vi "Interne Werte.vi"(0 "Regler Interne Werte":T2, 1 "Index":i32, 11 "error in (no error)":errorcluster caption="Fehler (Eingang, kein Fehler)", 12 "Aktionen Interne Werte":T1) -> (3 "Änderung?":bool, 4 "FT-IR":sgl[](array[numeric]), 6 "Ausgang":sgl[](array[numeric]), 8 "Dichtheitstest":sgl[](array[numeric]), 10 "Pumpe":sgl[](array[numeric]), 14 "error out":errorcluster caption="Fehler (Ausgang)", 15 "Druck Kalter Block":sgl[](array[numeric]))   [LabVIEW 2020, in "Regler.lvlib" / "Druckregler.lvlib"]
uses:
  Druckregler.lvlib
  Regler Interne Werte.ctl
  Aktionen Interne Werte.ctl
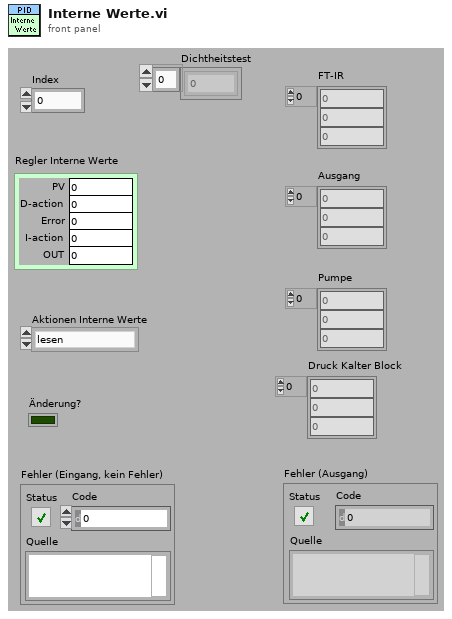
[diagram p1: front panel]
types:
  T1 = typedef "Regler.lvlib/Druckregler.lvlib/Aktionen Interne Werte.ctl" = enum16{"lesen", "FT-IR", "Ausgang", "Pumpe", "laden", "speichern", "Änderung?", "Druck Kalter Block", "Dichtheitstest"}
  T2 = typedef "Regler.lvlib/Druckregler.lvlib/Regler Interne Werte.ctl" = cluster{"PV":sgl, "D-action":sgl, "Error":sgl, "I-action":sgl, "OUT":sgl}
  T3 = cluster{sgl[][], sgl[][], sgl[][], sgl[][], sgl[][]}
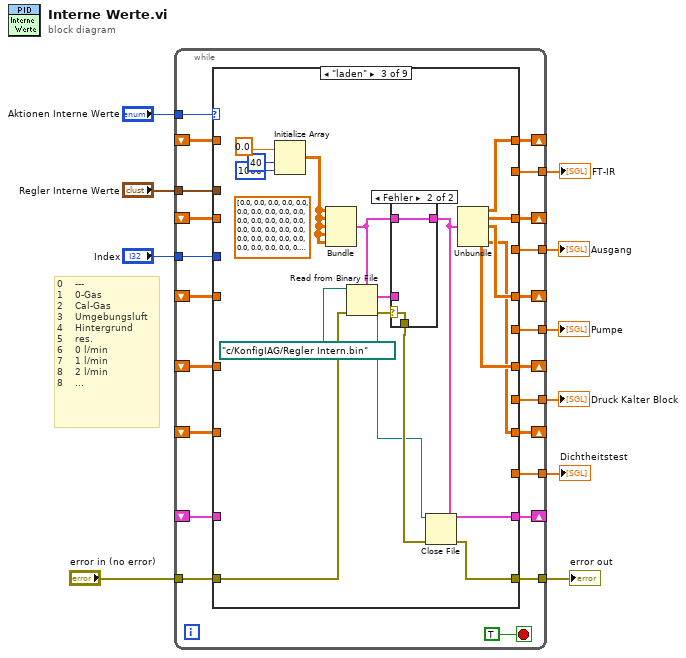
[diagram p0: block diagram]
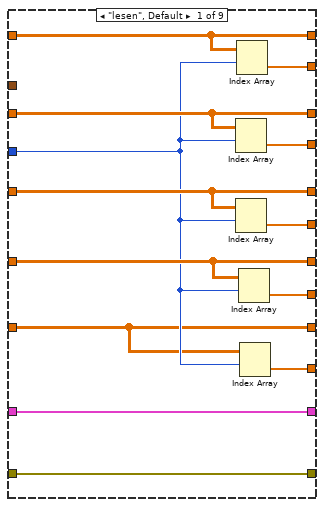
[diagram p2: hidden frame]
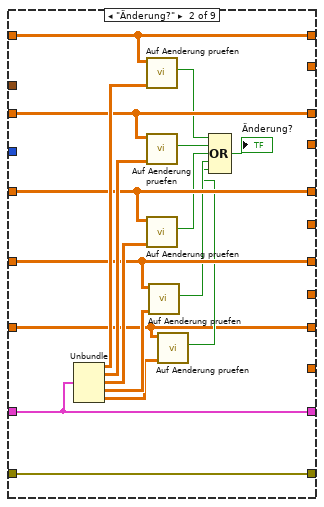
[diagram p3: hidden frame]
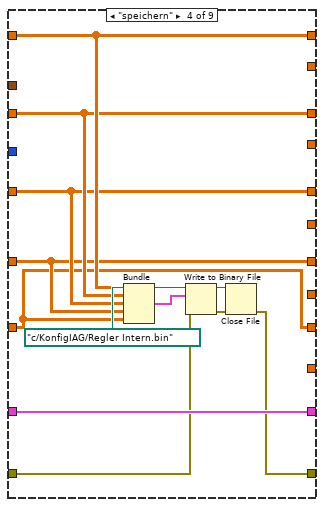
[diagram p5: hidden frame]
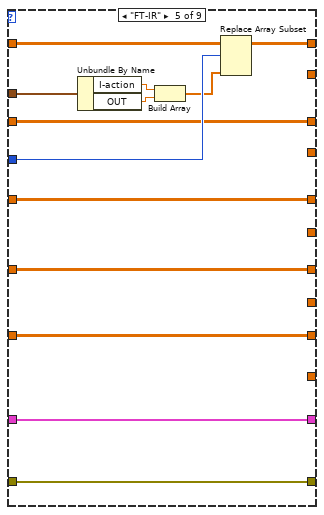
[diagram p6: hidden frame]
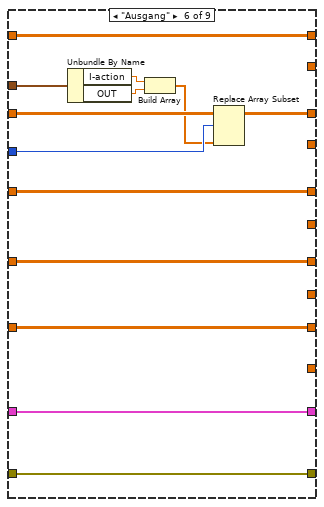
[diagram p7: hidden frame]
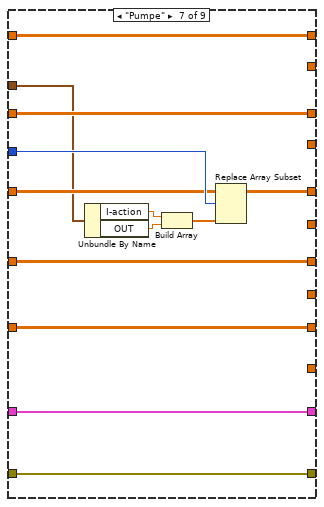
[diagram p8: hidden frame]
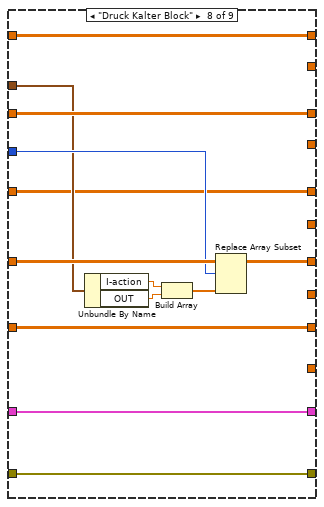
[diagram p9: hidden frame]
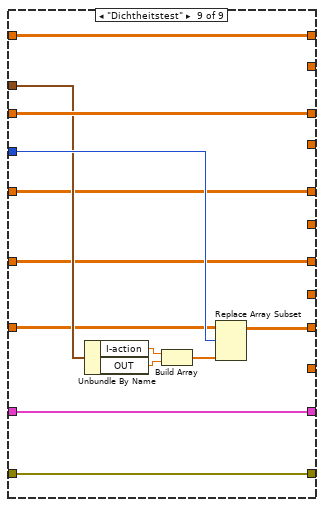
[diagram p10: hidden frame]
diagram:
  # "0    ---\n1    0-Gas\n2    Cal-Gas\n3    Umgebungsluft\n4    Hintergrund\n5    res.\n6    0 l/min\n7    1 l/min\n8    2 l/min\n8    ..."
  n1 = while {
    tunnel: "Aktionen Interne Werte" -> [w32]
    shift-right: [w31] -> _
    shift-left: _ -> [w25]
    shift-right: [w28] -> _
    shift-left: _ -> [w29]
    shift-right: [w26] -> _
    shift-left: _ -> [w27]
    tunnel: "Index" -> [w30]
    tunnel: "Regler Interne Werte" -> [w24]
    tunnel: [w23] -> w7
    tunnel: [w22] -> w6
    tunnel: [w21] -> w5
    shift-right: [w20] -> _
    shift-left: _ -> [w19]
    shift-right: [w17] -> _
    shift-left: _ -> [w16]
    tunnel: [w18] -> w4
    tunnel: "error in (no error)" -> [w15]
    tunnel: [w14] -> w2
    shift-right: [w13] -> _
    shift-left: _ -> [w12]
    tunnel: [w11] -> w1
    stop <- TRUE stop-if-true
    n2 = case shown="\"laden\"" w32 {
      tunnel: [w46 w63 w81 w96 w111 w121 w136 w150 w163] -> w31
      tunnel: w30 -> [w36 _ _ _ w110 w124 w137 w142 w157]
      tunnel: w29 -> [w45 w61 _ w95 w109 w123 w133 w149 w162]
      tunnel: [w45 w61 w80 w95 w109 w122 w133 w149 w162] -> w28
      tunnel: w27 -> [w44 w59 _ w94 w107 w120 w134 w140 w155]
      tunnel: [w44 w59 w79 w94 w107 w120 w135 w140 w155] -> w26
      tunnel: w25 -> [w46 w63 _ w96 w108 w121 w136 w150 w163]
      tunnel: w24 -> [_ _ _ _ w106 w117 w130 w141 w156]
      tunnel: [w43 _ _ _ _ _ _ _ _] -> w23
      tunnel: [w42 _ _ _ _ _ _ _ _] -> w22
      tunnel: [w41 _ _ _ _ _ _ _ _] -> w21
      tunnel: [w40 w64 w76 w93 w102 w115 w128 w148 w161] -> w20
      tunnel: w19 -> [w40 w64 _ w93 w102 w115 w128 w148 w161]
      tunnel: [w39 w52 w74 w92 w101 w114 w127 w143 w151] -> w17
      tunnel: [w38 _ _ _ _ _ _ _ _] -> w18
      tunnel: w16 -> [w39 w52 _ w92 w101 w114 w127 w144 w151]
      tunnel: w15 -> [w37 w50 w73 w91 w100 w113 w126 w139 w154]
      tunnel: [w37 w50 w70 w88 w100 w113 w126 w139 w154] -> w14
      tunnel: [w35 w47 w69 w87 w99 w112 w125 w138 w153] -> w13
      tunnel: w12 -> [w35 w47 _ w87 w99 w112 w125 w138 w152]
      tunnel: [w34 _ _ _ _ _ _ _ _] -> w11
      frame "lesen", Default {
        n3 = Index Array(array=w45, index (row)=w36) -> (element=w42:sgl[])  [unwired: 1 in]
        n4 = Index Array(array=w44, index (row)=w36) -> (element=w41:sgl[])  [unwired: 1 in]
        n5 = Index Array(array=w46, index (row)=w36) -> (element=w43:sgl[])  [unwired: 1 in]
        n6 = Index Array(array=w39, index (row)=w36) -> (element=w38:sgl[])  [unwired: 1 in]
        n7 = Index Array(array=w35, index (row)=w36) -> (element=w34:sgl[])  [unwired: 1 in]
      }
      frame "Änderung?" {
        n8 = Unbundle(w64) -> (w62:sgl[][], w60:sgl[][], w58:sgl[][], w53:sgl[][], w49:sgl[][])
        n9 = call "Auf Aenderung pruefen.vi"("Gespeicherte Werte"=w62, "Neue Werte"=w63) -> ("Änderung?"=w57:bool)  [unwired: 9 in]
        n10 = call "Auf Aenderung pruefen.vi"("Gespeicherte Werte"=w60, "Neue Werte"=w61) -> ("Änderung?"=w56:bool)  [unwired: 9 in]
        n11 = call "Auf Aenderung pruefen.vi"("Gespeicherte Werte"=w58, "Neue Werte"=w59) -> ("Änderung?"=w55:bool)  [unwired: 9 in]
        n12 = call "Auf Aenderung pruefen.vi"("Gespeicherte Werte"=w53, "Neue Werte"=w52) -> ("Änderung?"=w51:bool)  [unwired: 9 in]
        n13 = call "Auf Aenderung pruefen.vi"("Gespeicherte Werte"=w49, "Neue Werte"=w47) -> ("Änderung?"=w48:bool)  [unwired: 9 in]
        n14 = Compound Arithmetic op=OR(w57, w56, w55, w51, w48) -> (→"Änderung?":bool)
      }
      frame "laden" {
        (unwired) sgl[][] [[0.0, 0.0], [0.0, 0.0], [0.0, 0.0], [0.0, 0.0], [0.0, 0.0], [0.0, 0.0], [0.0, 0.0], [0.0, 0.0], [0.0, 0.0], [0.0, 0.0], [0.0, 0.0], [0.0, 0.0], [0.0, 0.0], [0.0, 0.0], [0.0, 0.0], [0.0, 0.0], [0.0, 0.0], [0.0, 0.0], [0.0, 0.0], [0.0, 0.0], [0.0, 0.0], [0.0, 0.0], [0.0, 0.0], [0.0, 0.0], [0.0, 0.0], [0.0, 0.0], [0.0, 0.0], [0.0, 0.0], [0.0, 0.0], [0.0, 0.0], [0.0, 0.0], [0.0, 0.0], [0.0, 0.0], [0.0, 0.0], [0.0, 0.0], [0.0, 0.0], [0.0, 0.0], [0.0, 0.0], [0.0, 0.0], [0.0, 0.0], [0.0, 0.0]] ("Angehängtes Array")
        n15 = Initialize Array(sgl 0.0 ("OUT"), 40 ("Dimension"), 1000 ("Dimension")) -> (w65:sgl[][])
        n16 = Bundle(w65, w65, w65, w65, w65) -> (w77:T3)  [unwired: 1 in]
        n17 = Read from Binary File(5:w77, 8:w73, 11:path "c:/KonfigIAG/Regler Intern.bin" ("Hinzugefügter Pfad")) -> (0:w75:errorcluster, 2:w78:T3, 3:w71:refnum<file>)  [unwired: 3 in, 1 out]
        n18 = case shown="Fehler" w75 {
          selector: w75 -> [w83 w85]
          tunnel: w78 -> [w84 _]
          tunnel: w77 -> [_ w86]
          tunnel: [w84 w86] -> w76
          tunnel: [w83 w85] -> w72
          frame No Error {
          }
          frame Error {
          }
        }
        n19 = Close File(refnum=w71, error in=w72) -> (error out=w70:errorcluster)  [unwired: 1 out]
        n20 = Unbundle(w76) -> (w81:sgl[][], w80:sgl[][], w79:sgl[][], w74:sgl[][], w69:sgl[][])
      }
      frame "speichern" {
        n21 = Bundle(w96, w95, w94, w92, w87) -> (w97:T3)  [unwired: 1 in]
        n22 = Write to Binary File(file (use dialog)=path "c:/KonfigIAG/Regler Intern.bin" ("Hinzugefügter Pfad"), data=w97, error in=w91) -> (refnum out=w89:refnum<file>, error out=w90:errorcluster)  [unwired: 4 out]
        n23 = Close File(refnum=w89, error in=w90) -> (error out=w88:errorcluster)  [unwired: 1 out]
      }
      frame "FT-IR" {
        n24 = Unbundle By Name(w106) -> ("I-action"=w104:sgl, "OUT"=w105:sgl)
        n25 = Build Array(w104, w105) -> (w103:sgl[])
        n26 = Replace Array Subset(array=w108, new element=w103, index (row)=w110) -> (w111:sgl[][])  [unwired: 1 in]
      }
      frame "Ausgang" {
        n27 = Unbundle By Name(w117) -> ("I-action"=w118:sgl, "OUT"=w119:sgl)
        n28 = Build Array(w118, w119) -> (w116:sgl[])
        n29 = Replace Array Subset(array=w123, new element=w116, index (row)=w124) -> (w122:sgl[][])  [unwired: 1 in]
      }
      frame "Pumpe" {
        n30 = Unbundle By Name(w130) -> ("I-action"=w131:sgl, "OUT"=w132:sgl)
        n31 = Build Array(w131, w132) -> (w129:sgl[])
        n32 = Replace Array Subset(array=w134, new element=w129, index (row)=w137) -> (w135:sgl[][])  [unwired: 1 in]
      }
      frame "Druck Kalter Block" {
        n33 = Unbundle By Name(w141) -> ("I-action"=w146:sgl, "OUT"=w145:sgl)
        n34 = Build Array(w146, w145) -> (w147:sgl[])
        n35 = Replace Array Subset(array=w144, new element=w147, index (row)=w142) -> (w143:sgl[][])  [unwired: 1 in]
      }
      frame "Dichtheitstest" {
        n36 = Unbundle By Name(w156) -> ("I-action"=w159:sgl, "OUT"=w158:sgl)
        n37 = Build Array(w159, w158) -> (w160:sgl[])
        n38 = Replace Array Subset(array=w152, new element=w160, index (row)=w157) -> (w153:sgl[][])  [unwired: 1 in]
      }
    }
  }
  "FT-IR" <- w7
  "Ausgang" <- w6
  "Pumpe" <- w5
  "Druck Kalter Block" <- w4
  "error out" <- w2
  "Dichtheitstest" <- w1
